vi "CalculateHighRateDeviceFeatures.vi"(8 "error in (no error)":errorcluster, 9 "Map in":T7, 10 "Waveforms":waveform(sgl)[](array[waveform]), 11 "Group in":T1) -> (0 "error out":errorcluster, 3 "Group out":T1)   [LabVIEW 2017, in "McsaAnalysisHighRate.lvlib"]
uses:
  <vilib>/addons/InsightCM/Devices/Shared/Mcsa/McsaAnalysisHighRate/McsaAnalysisHighRate.lvlib
  <vilib>/addons/PointValueMap/controls/PointMap.ctl
  <vilib>/addons/InsightCM/Devices/Shared/Mcsa/McsaAnalysisHighRate/controls/Group.ctl
  <vilib>/addons/InsightCM/Utilities/Analysis/MCSA/controls/McsaChannel.ctl
  <vilib>/addons/InsightCM/Utilities/Analysis/Shared/controls/Feature.ctl
  <vilib>/addons/InsightCM/Utilities/Analysis/Shared/controls/AmplitudeScale.ctl
  <vilib>/addons/InsightCM/MessageBus/Base/controls/KeyValuePair.ctl
  <vilib>/addons/InsightCM/Utilities/Analysis/MCSA/controls/McsaMotor.ctl
  <vilib>/addons/InsightCM/Utilities/Analysis/MCSA/McsaAnalysisFunctions.lvlib
  <vilib>/addons/PointValueMap/PointValueMap.lvlib
  <vilib>/addons/InsightCM/Utilities/Analysis/Shared/AnalysisHelper.lvlib
panel:
  out "Map out":T7
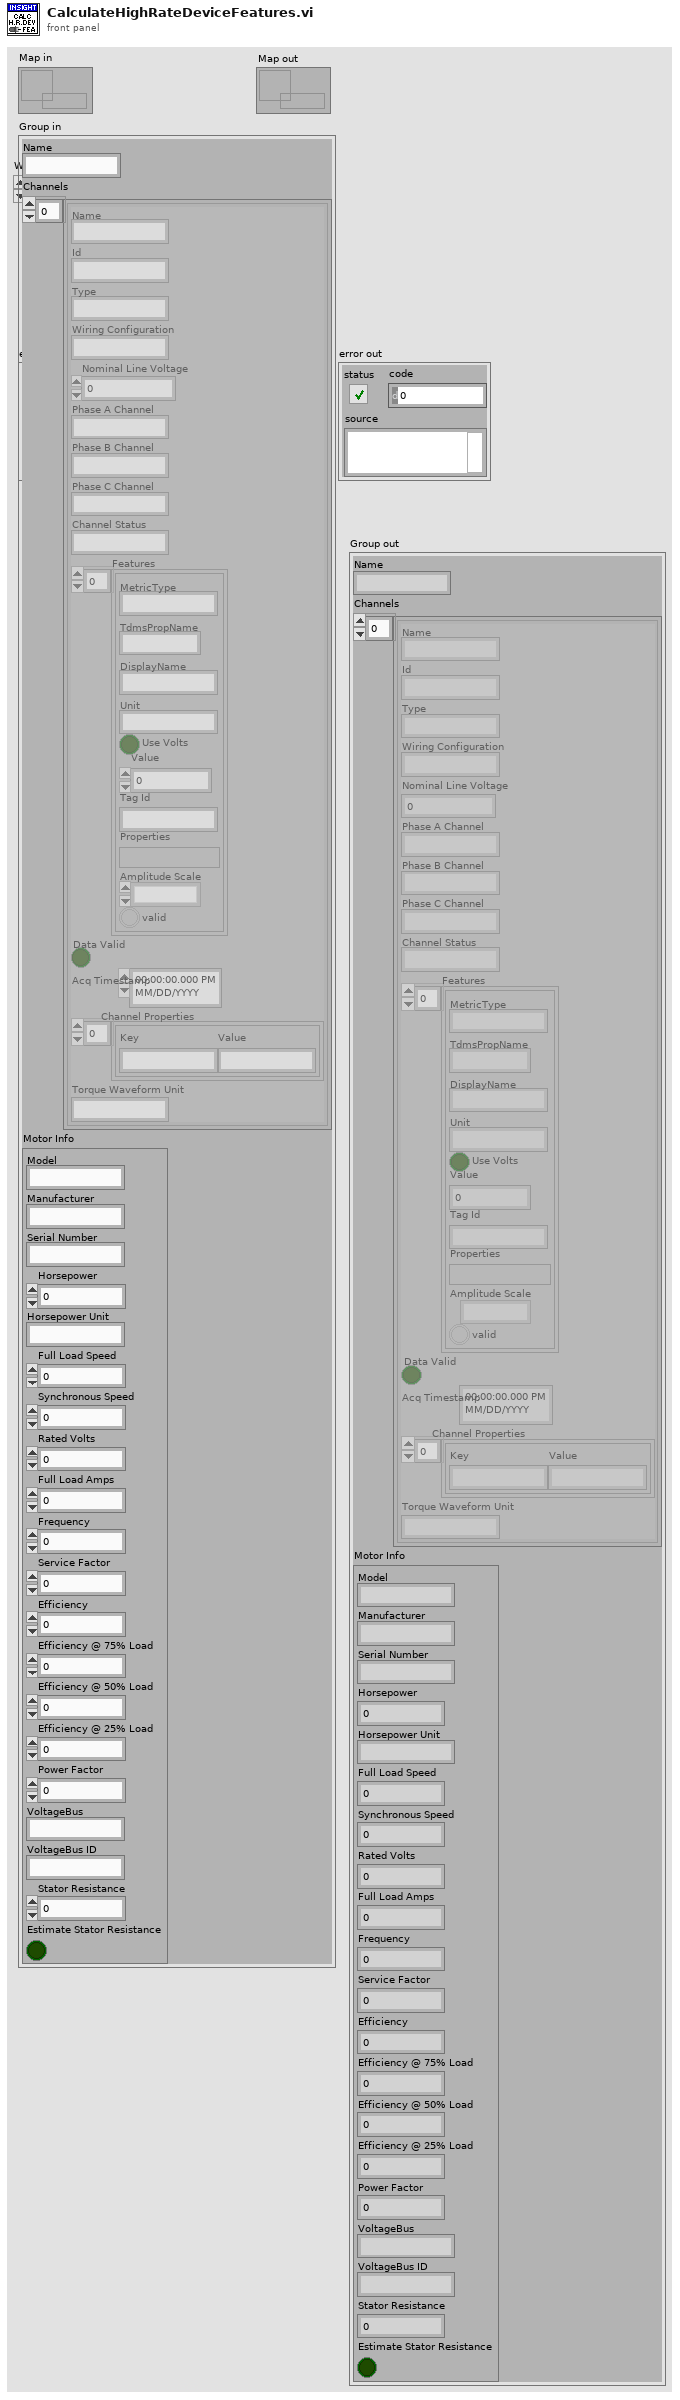
[diagram p1: front panel]
types:
  T1 = typedef "McsaAnalysisHighRate.lvlib/Group.ctl" = cluster{"Name":string, "Channels":T2[], "Motor Info":T6}
  T2 = typedef "McsaAnalysisFunctions.lvlib/McsaChannel.ctl" = cluster{"Name":string, "Id":string, "Type":string, "Wiring Configuration":string, "Nominal Line Voltage":dbl, "Phase A Channel":string, "Phase B Channel":string, "Phase C Channel":string, "Channel Status":string, "Features":T3[], "Data Valid":bool, "Acq Timestamp":timestamp, "Channel Properties":T5[], "Torque Waveform Unit":string}
  T3 = typedef "AnalysisHelper.lvlib/Feature.ctl" = cluster{"MetricType":string, "TdmsPropName":string, "DisplayName":string, "Unit":string, "Use Volts":bool, "Value":dbl, "Tag Id":string, "Properties":variant, "Amplitude Scale":T4, "valid":bool}
  T4 = typedef "AnalysisHelper.lvlib/AmplitudeScale.ctl" = enum16{"rms", "peak", "pk-pk"}
  T5 = typedef "KeyValuePair.ctl" = cluster{"Key":string, "Value":string}
  T6 = typedef "McsaAnalysisFunctions.lvlib/McsaMotor.ctl" = cluster{"Model":string, "Manufacturer":string, "Serial Number":string, "Horsepower":dbl, "Horsepower Unit":string, "Full Load Speed":dbl, "Synchronous Speed":dbl, "Rated Volts":dbl, "Full Load Amps":dbl, "Frequency":dbl, "Service Factor":dbl, "Efficiency":dbl, "Efficiency @ 75% Load":dbl, "Efficiency @ 50% Load":dbl, "Efficiency @ 25% Load":dbl, "Power Factor":dbl, "VoltageBus":string, "VoltageBus ID":string, "Stator Resistance":dbl, "Estimate Stator Resistance":bool}
  T7 = typedef "PointValueMap.lvlib/PointMap.ctl" = refnum<data-value>
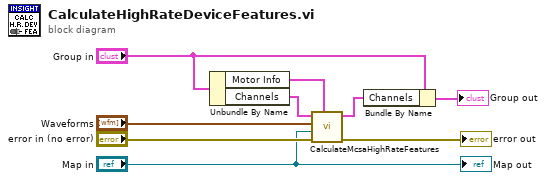
[diagram p0: block diagram]
diagram:
  n1 = Unbundle By Name("Group in") -> ("Motor Info"=w1:T6, "Channels"=w9:T2[])
  n2 = call <vilib>:"CalculateMcsaHighRateFeatures.vi"("motor informaiton"=w1, "error in (no error)"="error in (no error)", "Map"="Map in", "waveforms"="Waveforms", "channels"=w9) -> ("error out"=→"error out":errorcluster, "channels out"=w6:T2[])  [unwired: 5 in]
  n3 = Bundle By Name(cluster="Group in", "Channels"=w6) -> (→"Group out":T1)
  "Map out" <- "Map in"
